vi "test2.vi"() -> ()   [LabVIEW 2019]
panel:
  in  "stop":bool
  in  "Outlet 8":bool
  in  "Outlet 7":bool
  in  "Outlet 6":bool
  in  "Outlet 5":bool
  in  "Outlet 4":bool
  in  "Outlet 3":bool
  in  "Outlet 2":bool
  in  "Outlet 1":bool
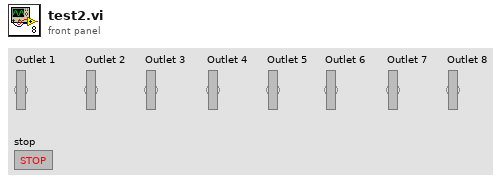
[diagram p1: front panel]
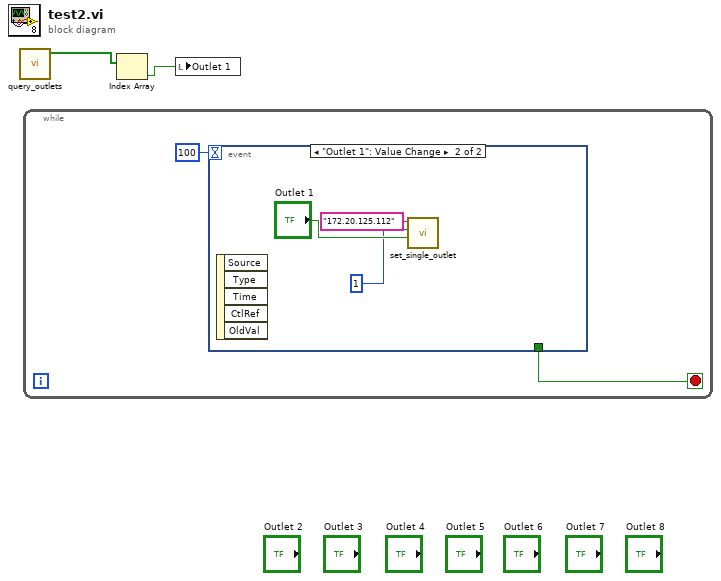
[diagram p0: block diagram]
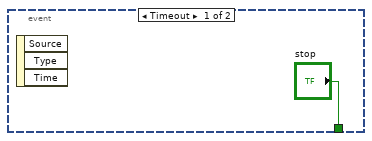
[diagram p2: hidden frame]
diagram:
  n1 = call "query_outlets.vi"() -> ("Switch status"=w2:bool[])  [unwired: 10 in, 1 out]
  n2 = while {
    stop <- w3 stop-if-true
    n3 = event shown="[1] \"Outlet 1\": Value Change" {
      selector: _ -> [_ _]
      dyn-events: _ -> [_ _]
      timeout: 100 -> [_ _]
      tunnel: ["stop" _] -> w3
      event Timeout {
        n4 = event-data() -> ()  [unwired: 1 in, 3 out]
      }
      event "Outlet 1": Value Change {
        n5 = event-data() -> ()  [unwired: 1 in, 5 out]
        n6 = call "set_single_outlet.vi"("Switch state"="Outlet 1", "Outlet #"=1, "IP / Hostname"="172.20.125.112") -> ()  [unwired: 9 in]
      }
    }
  }
  n7 = Index Array(array=w2) -> (element=w1:bool)  [unwired: 1 in]
  n8 = local write "Outlet 1"(w1) -> ()
